vi "Lock-in reference mode.vi"(8 "error in (no error)":errorcluster, 9 "read-only? (t)":bool=TRUE, 10 "set reference mode":enum16{"external", "internal"}(ring), 11 "VISA resource name":refnum<visa-resource-name>) -> (0 "error out":errorcluster, 2 "reference mode":string, 3 "VISA resource name out":refnum<visa-resource-name>)   [LabVIEW 2009, in "Lockin.lvclass"]
doc: "Sets and/or reads the current reference mode (internal or external) of the lock-in amplifier."
uses:
  Lockin.lvclass
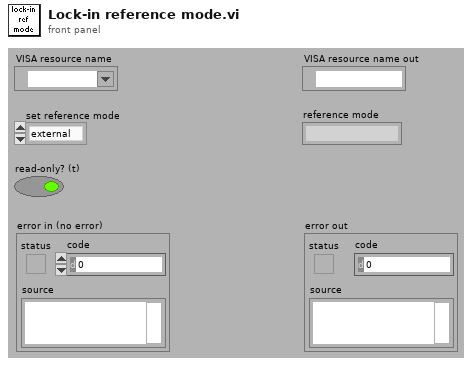
[diagram p1: front panel]
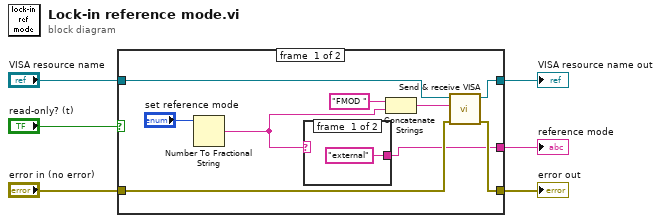
[diagram p0: block diagram]
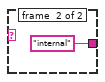
[diagram p2: hidden frame]
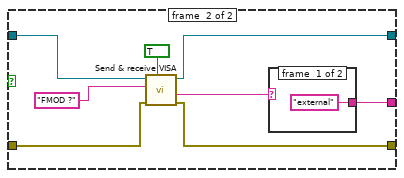
[diagram p3: hidden frame]
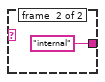
[diagram p4: hidden frame]
diagram:
  n1 = case shown="False" "read-only? (t)" {
    tunnel: "error in (no error)" -> [w13 w23]
    tunnel: [w12 w22] -> w4
    tunnel: "VISA resource name" -> [w11 w21]
    tunnel: [w10 w20] -> w2
    tunnel: [w7 w18] -> w1
    frame #0 {
      n2 = Number To Fractional String(number="set reference mode") -> (F-format string=w8:string)  [unwired: 3 out]
      n3 = case shown="\"0\"" w8 {
        tunnel: ["external" ("read buffer") "internal" ("read buffer")] -> w7
        frame #0 {
        }
        frame #1 {
        }
      }
      n4 = Concatenate Strings("FMOD " ("write buffer"), w8) -> (w14:string)
      n5 = call "Send & receive VISA.vi"("error in (no error)"=w13, "write buffer"=w14, "VISA resource name"=w11) -> ("error out"=w12:errorcluster, "VISA resource name out"=w10:refnum<visa-resource-name>)  [unwired: 2 in, 5 out]
    }
    frame #1 {
      n6 = call "Send & receive VISA.vi"("read? (f)"=TRUE, "error in (no error)"=w23, "write buffer"="FMOD ?", "VISA resource name"=w21) -> ("error out"=w22:errorcluster, "read buffer"=w19:string, "VISA resource name out"=w20:refnum<visa-resource-name>)  [unwired: 1 in, 4 out]
      n7 = case shown="\"0\"" w19 {
        tunnel: ["external" ("read buffer") "internal" ("read buffer")] -> w18
        frame #0 {
        }
        frame #1 {
        }
      }
    }
  }
  "error out" <- w4
  "VISA resource name out" <- w2
  "reference mode" <- w1
